vi "GA Init Look Ahead.vi"(8 "error in (no error)":errorcluster caption="错误输入（无错误）", 9 "plookAheadPara":T1, 10 "FifoIndex":i16, 11 "nCrdNum":i16) -> (0 "error out":errorcluster caption="错误输出", 1 "plookAheadPara out":T1, 3 "function return":i32)   [LabVIEW 2015, in "GAS.lvlib"]
doc: "extern \"C\" __declspec(dllimport) int GA_InitLookAhead(short nCrdNum,short FifoIndex,TLookAheadPrm* plookAheadPara);"
uses:
  <userlib>/BP_GAS/GAS.lvlib
  <userlib>/BP_GAS/GAS.dll
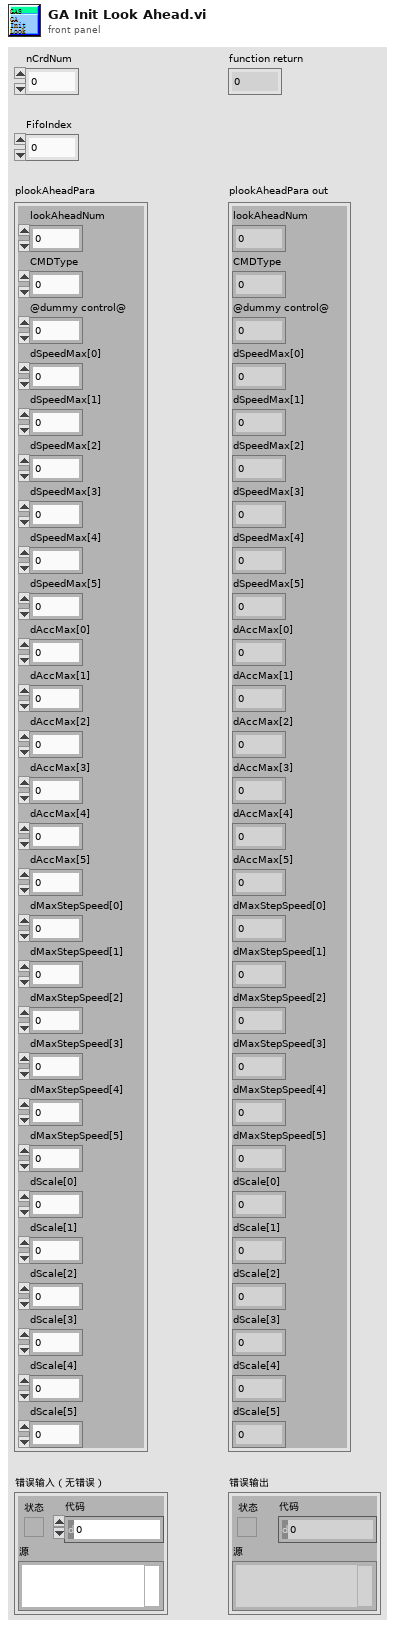
[diagram p1: front panel]
types:
  T1 = cluster{"lookAheadNum":i32, "CMDType":u8, "@dummy control@":i8, "dSpeedMax[0]":dbl, "dSpeedMax[1]":dbl, "dSpeedMax[2]":dbl, "dSpeedMax[3]":dbl, "dSpeedMax[4]":dbl, "dSpeedMax[5]":dbl, "dAccMax[0]":dbl, "dAccMax[1]":dbl, "dAccMax[2]":dbl, "dAccMax[3]":dbl, "dAccMax[4]":dbl, "dAccMax[5]":dbl, "dMaxStepSpeed[0]":dbl, "dMaxStepSpeed[1]":dbl, "dMaxStepSpeed[2]":dbl, "dMaxStepSpeed[3]":dbl, "dMaxStepSpeed[4]":dbl, "dMaxStepSpeed[5]":dbl, "dScale[0]":dbl, "dScale[1]":dbl, "dScale[2]":dbl, "dScale[3]":dbl, "dScale[4]":dbl, "dScale[5]":dbl}
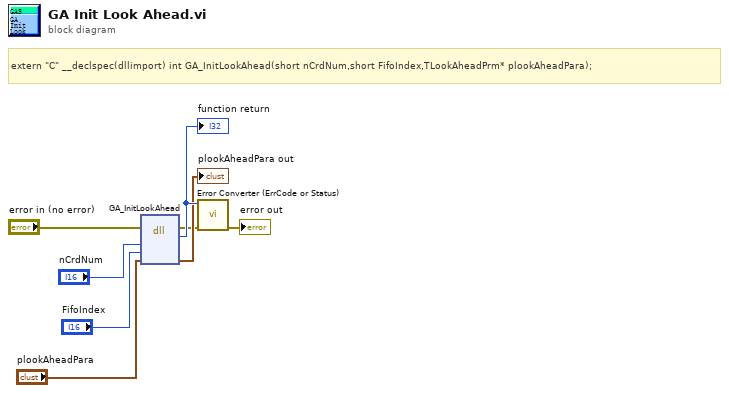
[diagram p0: block diagram]
diagram:
  # "extern \"C\" __declspec(dllimport) int GA_InitLookAhead(short nCrdNum,short FifoIndex,TLookAheadPrm* plookAheadPara);"
  n1 = dll-call lib="E:/Program Files (x86)/National Instruments/LabVIEW 2015/user.lib/BP_GAS/GAS.*" fn="GA_InitLookAhead"(error in="error in (no error)", "nCrdNum"="nCrdNum", "FifoIndex"="FifoIndex", "plookAheadPara"="plookAheadPara") -> (error out=w2:errorcluster, w8:i32, "plookAheadPara"=→"plookAheadPara out":T1)  [unwired: 4 in, 1 out]
  "function return" <- w8
  n2 = call "Error Converter (ErrCode or Status).vi"("error in (no error)"=w2, "error code"=w8) -> ("error out"=→"error out":errorcluster)  [unwired: 9 in]
